vi "Teleop.vi"(10 "Match Info":T1={"Autonomous Elapsed Seconds"=0.0, "TeleOp Elapsed Seconds"=0.0, "Disabled Elapsed Seconds"=0.0, "Visited Autonomous"=FALSE, "Visited TeleOp"=FALSE, "Visited Disabled"=FALSE, "Autonomous Settings"={"Autonomous Style"=enum."Independent", "VI Refnum"=refnum}}, 11 "Call Context":T2) -> ()   [LabVIEW 2016]
doc: "This VI is called for each TeleOp packet received from the DS where the robot is not disabled. It is often used to read from the joysticks and update I/O or to update setpoints for timed control loops. It should complete and return within 20 milliseconds or it may miss DS packets."
uses:
  <vilib>/Rock Robotics/WPI/DriverStation/WPI_DriverStationDerivedRobotMode.ctl
  <vilib>/Rock Robotics/WPI/DriverStation/WPI_DriverStationMatch Info.ctl
  <vilib>/Rock Robotics/WPI/Utilities/WPI_GetSetVariantRefNum.vi
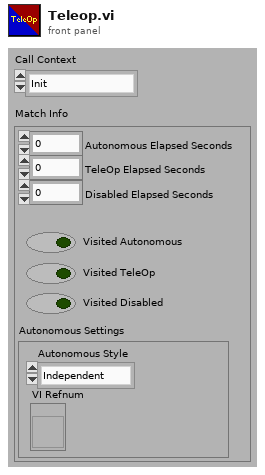
[diagram p1: front panel]
types:
  T1 = typedef "WPI_DriverStationMatch Info.ctl" = cluster{"Autonomous Elapsed Seconds":dbl, "TeleOp Elapsed Seconds":dbl, "Disabled Elapsed Seconds":dbl, "Visited Autonomous":bool, "Visited TeleOp":bool, "Visited Disabled":bool, "Autonomous Settings":cluster{"Autonomous Style":enum16{"Iterative", "Independent"}, "VI Refnum":refnum<vi>}}
  T2 = typedef "WPI_DriverStationDerivedRobotMode.ctl" = enum16{"Init", "Execute", "Stop"}
  T3 = typedef "WPI_JoystickDevRef.ctl" = cluster{"Device":T4}
  T4 = typedef "WPI_JoystickDeviceEnum.ctl" = enum16{"USB 0", "USB 1", "USB 2", "USB 3", "USB 4", "USB 5"}
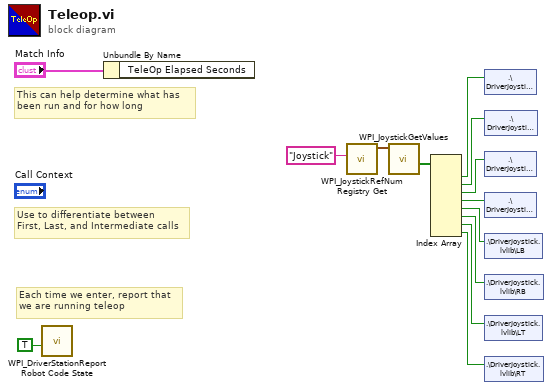
[diagram p0: block diagram]
diagram:
  # "Each time we enter, report that\nwe are running teleop"
  # "Use to differentiate between\nFirst, Last, and Intermediate calls"
  # "This can help determine what has\nbeen run and for how long"
  n1 = call <vilib>:"WPI_DriverStationReport Robot Code State.vi"("TeleOp"=TRUE ("Autonomous")) -> ()  [unwired: 10 in, 1 out]
  n2 = Unbundle By Name("Match Info") -> ()  [unwired: 1 out]
  n3 = call <vilib>:"WPI_JoystickRefNum Registry Get.vi"("refnum name"="Joystick") -> ("JoystickDevRef"=w10:T3)  [unwired: 9 in, 1 out]
  n4 = call <vilib>:"WPI_JoystickGetValues.vi"("JoystickDevRef"=w10) -> ("Buttons"=w9:bool[])  [unwired: 6 in, 4 out]
  n5 = Index Array(array=w9) -> (element #1=w8:bool, element #2=w7:bool, element #3=w6:bool, element #4=w5:bool, element #5=w4:bool, element #6=w3:bool, element #7=w2:bool, element #8=w1:bool)  [unwired: 8 in]
  n6 = shared-variable ".\\DriverJoystick.lvlib\\X"(w8) -> ()  [unwired: 1 in, 1 out]
  n7 = shared-variable ".\\DriverJoystick.lvlib\\A"(w7) -> ()  [unwired: 1 in, 1 out]
  n8 = shared-variable ".\\DriverJoystick.lvlib\\B"(w6) -> ()  [unwired: 1 in, 1 out]
  n9 = shared-variable ".\\DriverJoystick.lvlib\\Y"(w5) -> ()  [unwired: 1 in, 1 out]
  n10 = shared-variable ".\\DriverJoystick.lvlib\\LB"(w4) -> ()  [unwired: 1 in, 1 out]
  n11 = shared-variable ".\\DriverJoystick.lvlib\\RB"(w3) -> ()  [unwired: 1 in, 1 out]
  n12 = shared-variable ".\\DriverJoystick.lvlib\\LT"(w2) -> ()  [unwired: 1 in, 1 out]
  n13 = shared-variable ".\\DriverJoystick.lvlib\\RT"(w1) -> ()  [unwired: 1 in, 1 out]
